vi "voice_recognition.vi"() -> (1 "Maximum 3":dynamicdata(graph) caption="标准与输入信号的对比", 2 "标准信号":dynamicdata(graph), 3 "Maximum":dynamicdata(graph) caption="采集的语音信号", 4 "采集的语音信号":dynamicdata(graph), 6 "Maximum 2":dynamicdata(graph) caption="标准信号", 8 "Array 2":dbl[](array[numeric]) caption="输入信号", 10 "Array":dbl[](array[numeric]) caption="原始信号", 12 "x < y?":bool, 13 "布尔":bool, 14 "结果":dbl[](array[numeric]), 15 "amplitude":dbl caption="均值" format="%.2p")   [LabVIEW 2018]
uses:
  <vilib>/Analysis/baseanly.llb/Mean (DBL).vi
  <vilib>/express/express analysis/Spectral/Block/exnSpectralBlock spectral measurements power poly.vi
  <vilib>/express/express analysis/Spectral/Block/exnSpectralBlock spectral measurements power DDT.vi
  <vilib>/express/express analysis/Spectral/XNode/ExpressSpectralMeasurementsBlockNode.xnode
  <vilib>/express/express arith-compare/Formula/XNode/ExpressFormulaBlockNode.xnode
  <vilib>/Analysis/NI_AALBase.lvlib
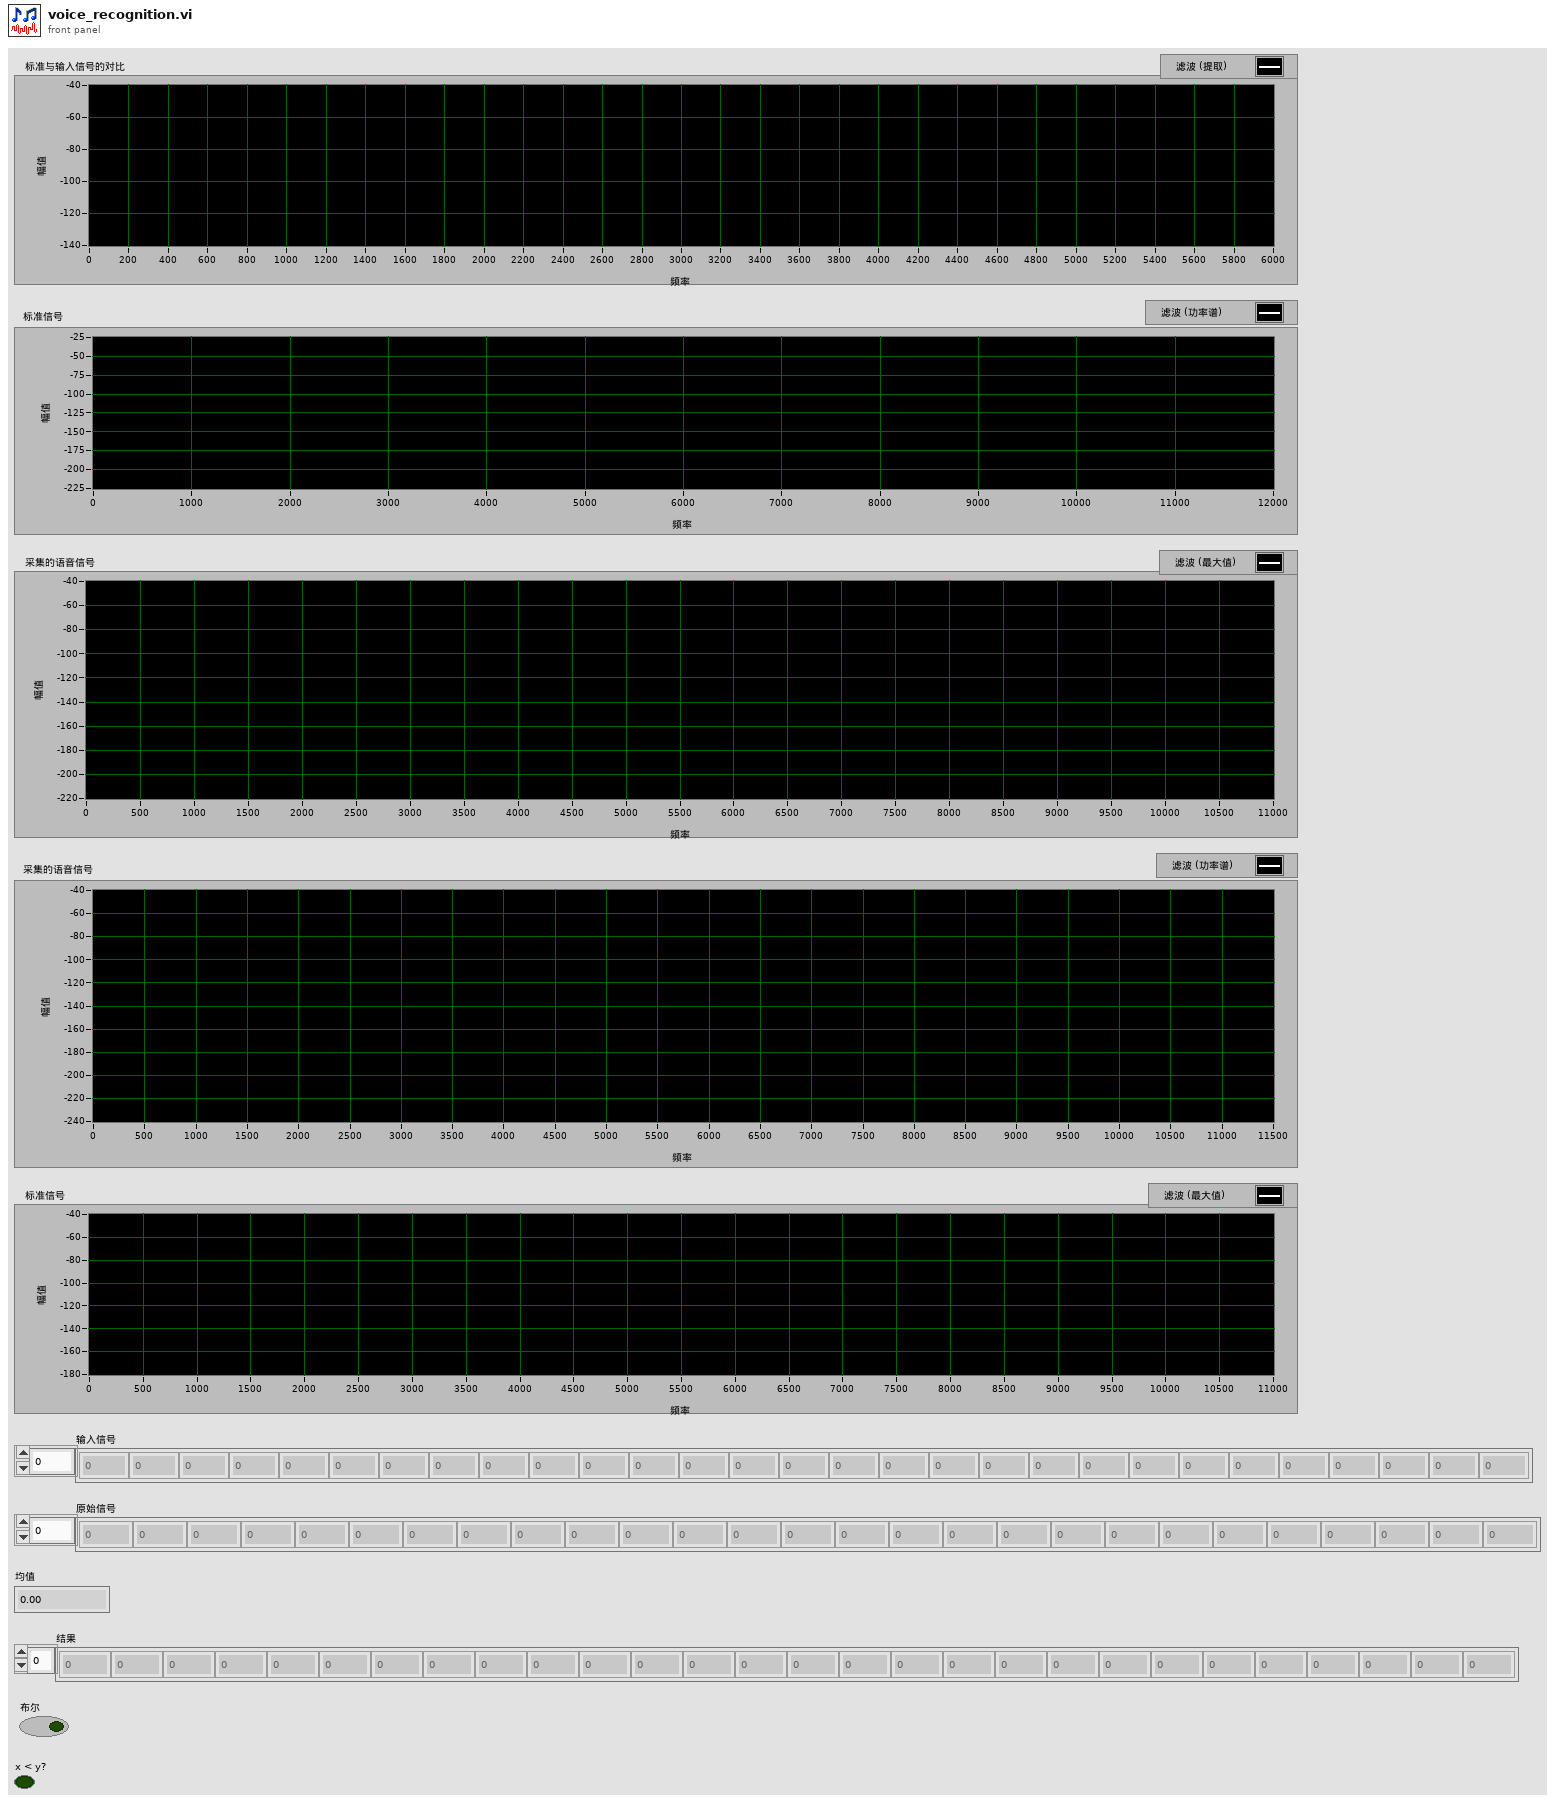
[diagram p1: front panel]
types:
  T1 = cluster{"averaging mode":u16, "weighting mode":u16, "number of averages":u32}
  T2 = cluster{"dB On (F)":bool, "unwrap phase (F)":bool, "convert to degree (F)":bool}
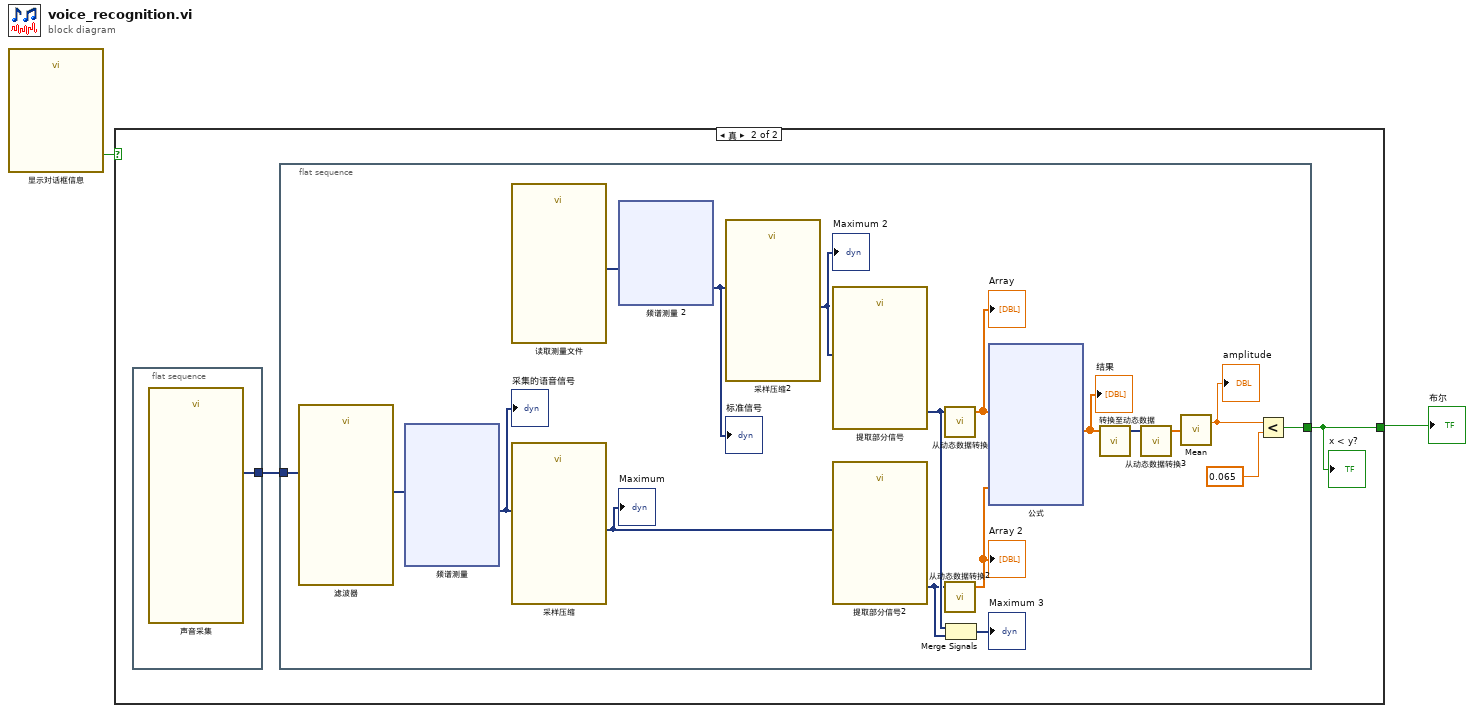
[diagram p0: block diagram]
diagram:
  n1 = call "显示对话框信息"() -> ("YES"=w1:bool)  [unwired: 10 in, 1 out]
  n2 = case shown="真" w1 {
    tunnel: [_ w3] -> w2
    frame False {
    }
    frame True {
      n3 = flat-sequence {
        tunnel: [w54] -> w4
        frame #0 {
          n4 = call "声音采集"() -> ("Data"=w54:dynamicdata)  [unwired: 18 in, 1 out]
        }
      }
      n5 = flat-sequence {
        tunnel: w4 -> [w22]
        tunnel: [w5] -> w3
        frame #0 {
          n6 = call "滤波器"("Signal"=w22) -> ("Filtered Signal"=w21:dynamicdata)  [unwired: 9 in, 1 out]
          n7 = xnode "频谱测量"("信号"=w21) -> ("功率谱"=w20:dynamicdata)  [unwired: 1 in, 1 out]
          "采集的语音信号" <- w20
          n8 = call "读取测量文件"() -> ("Signals"=w19:dynamicdata)  [unwired: 6 in, 5 out]
          n9 = call "采样压缩"("Signals"=w20) -> ("Maximum"=w15:dynamicdata)  [unwired: 8 in, 2 out]
          "Maximum" <- w15
          n10 = xnode "频谱测量 2"("信号"=w19) -> ("功率谱"=w18:dynamicdata)  [unwired: 1 in, 1 out]
          "标准信号" <- w18
          n11 = call "采样压缩2"("Signals"=w18) -> ("Maximum"=w16:dynamicdata)  [unwired: 8 in, 2 out]
          "Maximum 2" <- w16
          n12 = call "提取部分信号"("Signals"=w16) -> ("Section"=w14:dynamicdata)  [unwired: 9 in, 1 out]
          n13 = call "提取部分信号2"("Signals"=w15) -> ("Section"=w13:dynamicdata)  [unwired: 9 in, 1 out]
          n14 = call "从动态数据转换"("Dynamic Data Type"=w14) -> ("Array"=w12:dbl[])  [unwired: 3 in]
          "Array" <- w12
          n15 = call "从动态数据转换2"("Dynamic Data Type"=w13) -> ("Array"=w6:dbl[])  [unwired: 3 in]
          "Array 2" <- w6
          n16 = Merge Signals(w14, w13) -> (→"Maximum 3":dynamicdata)
          n17 = xnode "公式"("X1"=w12, "X2"=w6) -> ("结果"=w11:dbl[])  [unwired: 1 in, 1 out]
          "结果" <- w11
          n18 = call "转换至动态数据"("Array"=w11) -> ("Dynamic Data Type"=w10:dynamicdata)  [unwired: 3 in]
          n19 = call "从动态数据转换3"("Dynamic Data Type"=w10) -> ("Array"=w9:dbl[])  [unwired: 3 in]
          n20 = call-poly <vilib>:"Mean.vi"("X"=w9) -> ("mean"=w7:dbl)  [unwired: 1 out]
          "amplitude" <- w7
          n21 = Less?(x=w7, y=0.065 ("数值")) -> (x < y?=w5:bool)
        }
      }
      "x < y?" <- w3
    }
  }
  "布尔" <- w2
